vi "LV DLL 2.vi"(1 "Boolean":bool, 2 "Array":dbl[](array[numeric]) format="%.2f", 3 "String":string, 4 "Numeric":dbl format="%.2f") -> (0 "output Cluster":T1 {"Array" format="%.2f"; "Numeric" format="%.2f"})   [LabVIEW 2012]
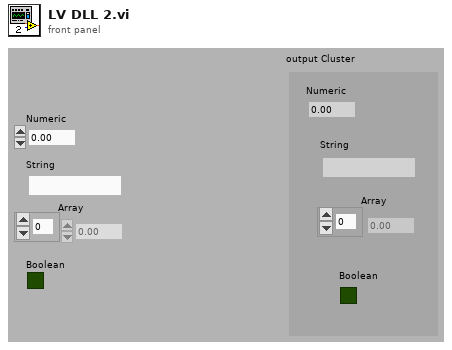
[diagram p1: front panel]
types:
  T1 = cluster{"Numeric":dbl, "String":string, "Array":dbl[], "Boolean":bool}
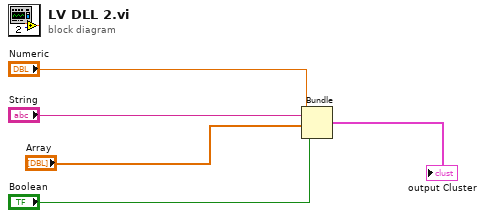
[diagram p0: block diagram]
diagram:
  n1 = Bundle("Numeric"="Numeric", "String"="String", "Array"="Array", "Boolean"="Boolean") -> (→"output Cluster":T1)  [unwired: 1 out]
